vi "PH_Beamline.Calc State.vi"(0 "i ref in":refnum<vi>, 5 "error in (no error)":errorcluster) -> (14 "i ref out":refnum<vi>, 19 "error out":errorcluster)   [LabVIEW 2014, in "PH_Beamline.lvlib"]
doc: "This VI contains all the VIs necesarry to calculate the state of all the subsystems and finally to derive the sum signal."
uses:
  PH_Beamline.lvlib
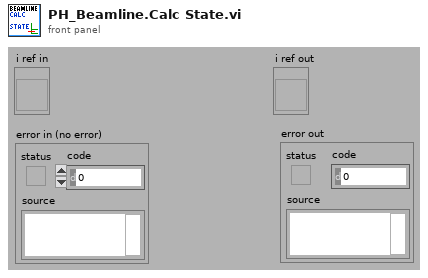
[diagram p1: front panel]
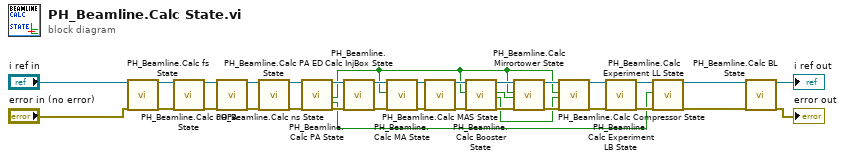
[diagram p0: block diagram]
diagram:
  n1 = call "PH_Beamline.Calc fs State.vi"("i ref in"="i ref in", "error in (no error)"="error in (no error)") -> ("i ref out"=w2:refnum<vi>, "error out"=w26:errorcluster)  [unwired: 16 in]
  n2 = call "PH_Beamline.Calc uOPA State.vi"("i ref in"=w2, "error in (no error)"=w26) -> ("i ref out"=w1:refnum<vi>, "error out"=w3:errorcluster)  [unwired: 16 in]
  n3 = call "PH_Beamline.Calc ns State.vi"("i ref in"=w1, "error in (no error)"=w3) -> ("i ref out"=w25:refnum<vi>, "error out"=w23:errorcluster)  [unwired: 16 in]
  n4 = call "PH_Beamline.Calc PA ED State.vi"("i ref in"=w25, "error in (no error)"=w23) -> ("i ref out"=w24:refnum<vi>, "error out"=w22:errorcluster)  [unwired: 16 in]
  n5 = call "PH_Beamline.Calc PA State.vi"("i ref in"=w24, "error in (no error)"=w22) -> ("i ref out"=w32:refnum<vi>, "PA Exit closed or shining into LL"=w5:bool, "PA Exit closed"=w4:bool, "error out"=w30:errorcluster)  [unwired: 14 in]
  n6 = call "PH_Beamline.Calc InjBox State.vi"("i ref in"=w32, "error in (no error)"=w30) -> ("i ref out"=w31:refnum<vi>, "error out"=w29:errorcluster)  [unwired: 16 in]
  n7 = call "PH_Beamline.Calc MA State.vi"("i ref in"=w31, "PA Exit closed or shining into LL"=w5, "error in (no error)"=w29) -> ("i ref out"=w21:refnum<vi>, "error out"=w19:errorcluster)  [unwired: 15 in]
  n8 = call "PH_Beamline.Calc MAS State.vi"("i ref in"=w21, "error in (no error)"=w19) -> ("i ref out"=w20:refnum<vi>, "error out"=w18:errorcluster)  [unwired: 16 in]
  n9 = call "PH_Beamline.Calc Booster State.vi"("i ref in"=w20, "PA Exit closed or shining into LL"=w5, "error in (no error)"=w18) -> ("i ref out"=w33:refnum<vi>, "Not shining to Mirrortower"=w7:bool, "Not shining Experiment LB"=w6:bool, "error out"=w34:errorcluster)  [unwired: 13 in]
  n10 = call "PH_Beamline.Calc Mirrortower State.vi"("i ref in"=w33, "PA Exit closed or shining into LL"=w5, "Not shining to Mirrortower"=w7, "error in (no error)"=w34) -> ("i ref out"=w15:refnum<vi>, "error out"=w14:errorcluster)  [unwired: 14 in]
  n11 = call "PH_Beamline.Calc Compressor State.vi"("i ref in"=w15, "PA Exit closed or shining into LL"=w5, "Not shining Experiment LB"=w6, "error in (no error)"=w14) -> ("i ref out"=w13:refnum<vi>, "error out"=w12:errorcluster)  [unwired: 14 in]
  n12 = call "PH_Beamline.Calc Experiment LB State.vi"("i ref in"=w13, "error in (no error)"=w12) -> ("i ref out"=w10:refnum<vi>, "error out"=w11:errorcluster)  [unwired: 16 in]
  n13 = call "PH_Beamline.Calc Experiment LL State.vi"("i ref in"=w10, "PA Exit closed"=w4, "error in (no error)"=w11) -> ("i ref out"=w9:refnum<vi>, "error out"=w8:errorcluster)  [unwired: 15 in]
  n14 = call "PH_Beamline.Calc BL State.vi"("i ref in"=w9, "error in (nop error)"=w8) -> ("i ref out"=→"i ref out":refnum<vi>, "error out"=→"error out":errorcluster)  [unwired: 16 in]
